vi "disable_ui.vi"(11 "UI":T1) -> ()   [LabVIEW 2017]
uses:
  ui.ctl
  classes/dc_power_supply/DC_power_supply.lvclass
  classes/report/Report.lvclass
  ui_buttons.ctl
  types/boc_type.ctl
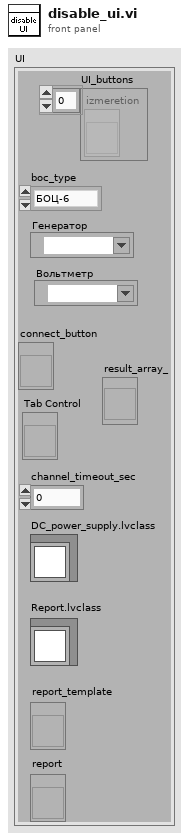
[diagram p1: front panel]
types:
  T1 = typedef "ui.ctl" = cluster{"UI_buttons":T2, "Tab Control":refnum<vi>, "connect_button":refnum<vi>, "generator":refnum<visa-resource-name>, "voltmetr":refnum<visa-resource-name>, "channel_timeout_sec":dbl, "boc_type":T3, "result_array_":refnum<vi>, "DC_power_supply.lvclass":refnum<class "DC_power_supply.lvclass">, "Report.lvclass":refnum<class "Report.lvclass">, "report_template":refnum<vi>, "report":refnum<vi>}
  T2 = typedef "ui_buttons.ctl" = refnum<vi>[]
  T3 = typedef "boc_type.ctl" = enum16{"БОЦ-6", "БОЦ-12"}
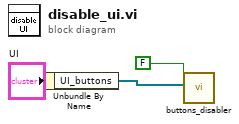
[diagram p0: block diagram]
diagram:
  n1 = Unbundle By Name("UI") -> ("UI_buttons"=w1:T2)
  n2 = call "buttons_disabler.vi"("Array"=w1, "s"=FALSE) -> ()  [unwired: 10 in]
